vi "AdressIC2NumConv.vi"(11 "Cluster":cluster{string, string, string}) -> (0 "NofBytes":u8, 3 "Address":u8)   [LabVIEW 2017, in "ArduinoLib.lvlib"]
uses:
  ArduinoLib.lvlib
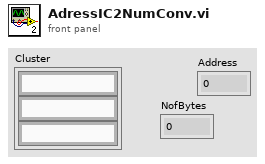
[diagram p1: front panel]
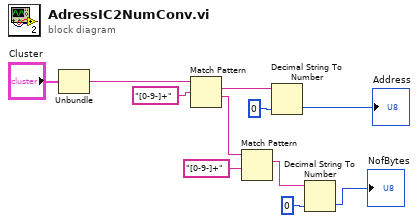
[diagram p0: block diagram]
diagram:
  n1 = Unbundle("Cluster") -> (w9:string)  [unwired: 2 out]
  n2 = Match Pattern(string=w9, regular expression="[0-9-]+") -> (match substring=w7:string, after substring=w5:string)  [unwired: 1 in, 2 out]
  n3 = Match Pattern(string=w5, regular expression="[0-9-]+") -> (match substring=w2:string)  [unwired: 1 in, 3 out]
  n4 = Decimal String To Number(string=w7, default (0L)=u8 0 ("default (0 I32)")) -> (number=→"Address":u8)  [unwired: 1 in, 1 out]
  n5 = Decimal String To Number(string=w2, default (0L)=u8 0 ("default (0 I32)")) -> (number=→"NofBytes":u8)  [unwired: 1 in, 1 out]
